vi "Stop WiFi Hotspot.vi"() -> (0 "error out":errorcluster, 1 "standard error":string, 2 "return code":i32)   [LabVIEW 2015]
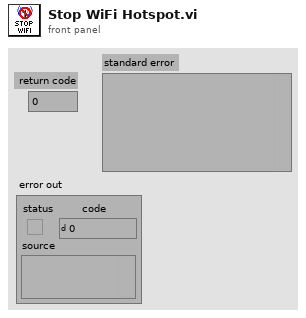
[diagram p1: front panel]
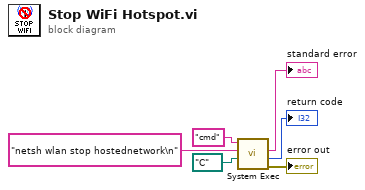
[diagram p0: block diagram]
diagram:
  n1 = call <vilib>:"System Exec.vi"("working directory"=path "C:/", "standard input"="netsh wlan stop hostednetwork\n" ("format string"), "command line"="cmd") -> ("error out"=→"error out":errorcluster, "return code"=→"return code":i32, "standard error"=→"standard error":string)  [unwired: 5 in, 1 out]
